vi "RSZVB Set RGB Color.vi"(4 "Green (0)":dbl format="%^.3e", 5 "Trace Width (1)":i32=1, 6 "Trace Style (0: Solid)":i32(ring) items=["Solid", "Dashed", "Dotted", "DDotted", "DDDotted"], 7 "Blue (0)":dbl format="%^.3e", 8 "error in (no error)":errorcluster {"code" format="%.0x"}, 9 "Red (0)":dbl format="%^.3e", 10 "Element (1: Background)":i32(ring)=1 items=["Background"=1, "Text"=2, "Selected Text"=3, "Grid"=4, "Reference Line"=5, "Same Color for all Markers"=0, "Horizontal Line / Vertical Range Lines"=7, "Diagram Title"=8, "Limit Fail Trace Color"=9, "Limit Line Type Off"=10, "Limit Line Type Upper"=11, "Limit Line Type Lower"=12, "Trace 1"=13, "Trace 2"=14, "Trace 3"=15, "Trace 4"=16, "Trace 5"=17, "Trace 6"=18, "Trace 7"=19, "Trace 8"=20, "Trace 9"=21, "Trace 10"=22, "Trace 11"=23, "Trace 12"=24, "Trace 13"=25, "Trace 14"=26, "Trace 15"=27, "Trace 16"=28], 11 "VISA session":refnum<visa-resource-name>) -> (0 "error out":errorcluster {"code" format="%.0x"}, 3 "dup VISA session":refnum<visa-resource-name>)   [LabVIEW 2011]
doc: "This VI defines the color of all display elements based on the Red/Green/Blue color model.\n\nRemote-control command(s):\nDISPlay:CMAP<Element>:RGB <red>, <green>, <blue> [,<trace_style>, <trace_width>]"
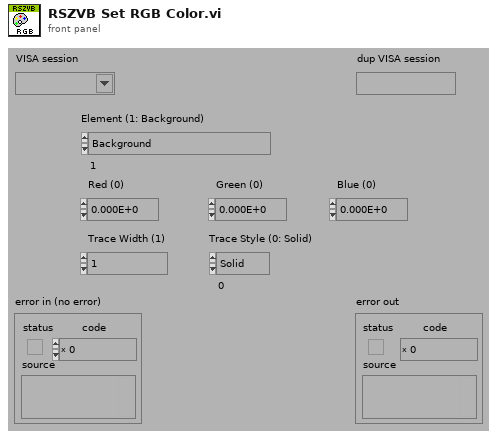
[diagram p1: front panel]
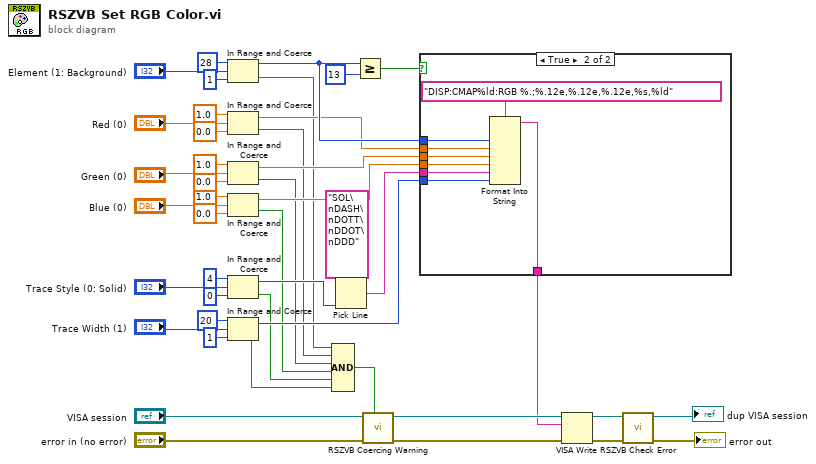
[diagram p0: block diagram]
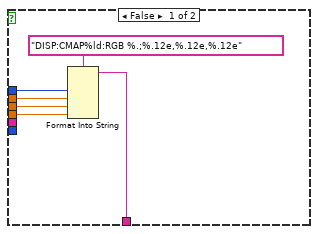
[diagram p2: hidden frame]
diagram:
  n1 = In Range and Coerce(upper limit=28, x="Element (1: Background)", lower limit=1) -> (coerced(x)=w15:i32, In Range?=w7:bool)
  n2 = In Range and Coerce(upper limit=1.0, x="Red (0)", lower limit=0.0) -> (coerced(x)=w14:dbl, In Range?=w6:bool)
  n3 = In Range and Coerce(upper limit=1.0, x="Green (0)", lower limit=0.0) -> (coerced(x)=w13:dbl, In Range?=w5:bool)
  n4 = In Range and Coerce(upper limit=1.0, x="Blue (0)", lower limit=0.0) -> (coerced(x)=w12:dbl, In Range?=w4:bool)
  n5 = In Range and Coerce(upper limit=4, x="Trace Style (0: Solid)", lower limit=0) -> (coerced(x)=w10:i32, In Range?=w3:bool)
  n6 = In Range and Coerce(upper limit=20, x="Trace Width (1)", lower limit=1) -> (coerced(x)=w8:i32, In Range?=w2:bool)
  n7 = Compound Arithmetic op=AND(w7, w6, w5, w4, w3, w2) -> (w42:bool)
  n8 = Pick Line(multi-line string="SOL\nDASH\nDOTT\nDDOT\nDDD", line index=w10) -> (output string=w9:string)  [unwired: 1 in]
  n9 = Greater Or Equal?(x=w15, y=13) -> (x >= y?=w16:bool)
  n10 = call "RSZVB Coercing Warning.vi"("In Range?"=w42, "error in (no error)"="error in (no error)", "VISA session"="VISA session") -> ("error out"=w41:errorcluster, "dup VISA session"=w40:refnum<visa-resource-name>)  [unwired: 7 in]
  n11 = case shown="True" w16 {
    tunnel: w15 -> [w49 w57]
    tunnel: w14 -> [w48 w56]
    tunnel: w13 -> [w47 w55]
    tunnel: w12 -> [w46 w54]
    tunnel: [w45 w53] -> w1
    tunnel: w9 -> [_ w52]
    tunnel: w8 -> [_ w51]
    frame False {
      n12 = Format Into String(format string="DISP:CMAP%ld:RGB %.;%.12e,%.12e,%.12e", w49, w48, w47, w46) -> (resulting string=w45:string)  [unwired: 2 in, 1 out]
    }
    frame True {
      n13 = Format Into String(format string="DISP:CMAP%ld:RGB %.;%.12e,%.12e,%.12e,%s,%ld", w57, w56, w55, w54, w52, w51) -> (resulting string=w53:string)  [unwired: 2 in, 1 out]
    }
  }
  n14 = VISA Write(VISA resource name=w40, write buffer=w1, error in (no error)=w41) -> (VISA resource name out=w44:refnum<visa-resource-name>, error out=w43:errorcluster)  [unwired: 1 out]
  n15 = call "RSZVB Check Error.vi"("error in (no error)"=w43, "VISA session"=w44) -> ("error out"=→"error out":errorcluster, "dup VISA session"=→"dup VISA session":refnum<visa-resource-name>)  [unwired: 8 in]
